vi "gentec-M-Link.Set Trigger Level.vi"(0 "VISA resource In":refnum<visa-resource-name>, 2 "Trigger Level [%]":dbl=10.0, 5 "error in (no error)":errorcluster) -> (11 "Data Read":string, 13 "Read Timeout":bool, 14 "VISA resource Out":refnum<visa-resource-name>, 16 "Success":bool, 19 "error out":errorcluster)   [LabVIEW 2014, in "gentec-M-Link - Driver.lvlib"]
doc: "Data to write: trg<n> where <n> is a number\n\nSets the instrument trigger level in %. Replies ok."
uses:
  gentec-M-Link - Driver.lvlib
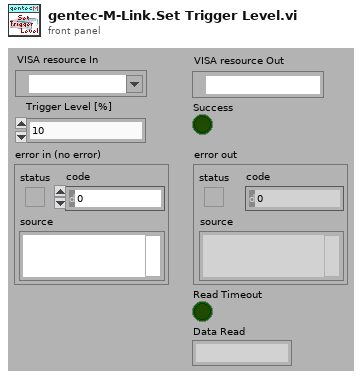
[diagram p1: front panel]
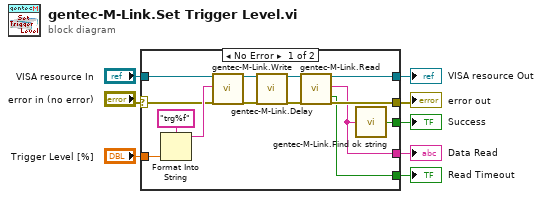
[diagram p0: block diagram]
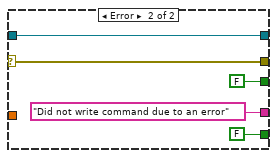
[diagram p2: hidden frame]
diagram:
  n1 = case shown="No Error" "error in (no error)" {
    selector: "error in (no error)" -> [w18 w27]
    tunnel: [w20 w27] -> w7
    tunnel: "Trigger Level [%]" -> [w19 _]
    tunnel: "VISA resource In" -> [w17 w26]
    tunnel: [w15 FALSE ("Found")] -> w4
    tunnel: [w14 w26] -> w3
    tunnel: [w13 FALSE ("Read Timeout")] -> w1
    tunnel: [w12 "Did not write command due to an error" ("Data Read")] -> w2
    frame No Error {
      n2 = Format Into String(format string="trg%f", w19) -> (resulting string=w21:string)  [unwired: 2 in, 1 out]
      n3 = call "gentec-M-Link.Write.vi"("VISA resource (In)"=w17, "Data To Write"=w21, "error in (no error)"=w18) -> ("VISA resource (Out)"=w10:refnum<visa-resource-name>, "error out"=w16:errorcluster)  [unwired: 14 in, 1 out]
      n4 = call "gentec-M-Link.Delay.vi"("VISA resource In"=w10, "error in (no error)"=w16) -> ("VISA resource Out"=w9:refnum<visa-resource-name>, "error out"=w11:errorcluster)  [unwired: 16 in]
      n5 = call "gentec-M-Link.Read.vi"("VISA resource (In)"=w9, "error in (no error)"=w11) -> ("VISA resource (Out)"=w14:refnum<visa-resource-name>, "Data Read"=w12:string, "Read Timeout"=w13:bool, "error out"=w20:errorcluster)  [unwired: 13 in, 1 out]
      n6 = call "gentec-M-Link.Find ok string.vi"("string"=w12) -> ("Found"=w15:bool)
    }
    frame Error {
    }
  }
  "error out" <- w7
  "Success" <- w4
  "VISA resource Out" <- w3
  "Data Read" <- w2
  "Read Timeout" <- w1
